vi "Create_Element_List.vi"() -> (0 "Current Element":T2, 1 "Element List":T1(array[cluster]))   [LabVIEW 2009]
panel:
  in  "String":string
  in  "Charakters_Cluster":T3={"Initial position"=[24.39, -7.31], "interval of charactors (Y)\n\"-\"down; \"+\" up"=0.0, "interval of charactors (X)\n\"-\" right; \"+\" left"=-0.7, "change size factor\nheight=1mm*factor\nwidth=0.5mm*factor"=1.0, "String of machining charactors"="", "XY Line Arc trj"={"Velocity (units/s)"=3.0, "Acceleration (unts/s2)"=50.0, "Number of times of execution"=1}} {"XY Line Arc trj"."Acceleration (unts/s2)" format="%.6f"; "XY Line Arc trj"."Velocity (units/s)" format="%.6f"; "XY Line Arc trj"."Number of times of execution" format="%.6f"; "Initial position" format="%.6f"}
  in  "Elektrode_Hole_Cluster":T4={"IR"=0.0, "Center of the hole  from left edge"=9.9, "Center of the hole from bottom edge"=2.35, "OR"=0.4, "ablation rate"=0.01, "change of radus"=0.01, "Depth of the hole"=4.0, "XY Line Arc Trajectory"={"Velocity (units/s)"=0.5, "Acceleration (unts/s2)"=20.0, "Number of times of execution"=1}} {"XY Line Arc Trajectory"."Acceleration (unts/s2)" format="%.6f"; "XY Line Arc Trajectory"."Velocity (units/s)" format="%.6f"; "XY Line Arc Trajectory"."Number of times of execution" format="%.6f"}
  in  "Gas_Jet_Cluster":T5={"Hight to groove(tube center)"=3.0, "Origin to jet outlet (Jet toal)"=10.0, "Laser interval tube"=0.01, "Ab rate tube"=0.016, "Machining geometry (mm)"={"a0 radius"=0.35, "a0 depth"=0.5, "b0 radius"=0.1, "b0(depth)"=0.15, "a1 radius"=0.2, "a1 depth"=0.3}, "Gap between  \nl1 and l2 "=0.003, "Length"={" l0"=0.5, "l1"=0.35, "l 2"=0.5, "l 3"=0.5}, "Laser interval jet"=0.008, "Ab rate jet"=0.01, "XY Line Arc Trajectory jet"={"Velocity (units/s)"=3.0, "Acceleration (unts/s2)"=20.0, "Number of times of execution"=1}, "XY Line Arc Trajectory tube"={"Velocity (units/s)"=3.0, "Acceleration (unts/s2)"=20.0, "Number of times of execution"=1}} {"XY Line Arc Trajectory tube"."Acceleration (unts/s2)" format="%.6f"; "XY Line Arc Trajectory tube"."Velocity (units/s)" format="%.6f"; "XY Line Arc Trajectory tube"."Number of times of execution" format="%.6f"; "XY Line Arc Trajectory jet"."Acceleration (unts/s2)" format="%.6f"; "XY Line Arc Trajectory jet"."Velocity (units/s)" format="%.6f"; "XY Line Arc Trajectory jet"."Number of times of execution" format="%.6f"}
  in  "Curved_Slot_Cluster":T6={"X distance from left edge"=10.5, "Height to groove"=2.5, "Remove distance"=3.5, "a0 radius"=0.9, "ablation rate"=0.01, "interval between laser path"=0.01, "Length "=11.0, "XY Line Arc Trajectory part 1"={"Velocity (units/s)"=3.0, "Acceleration (unts/s2)"=20.0, "Number of times of execution"=1}, "Slot geometry"={FALSE, FALSE}} {"XY Line Arc Trajectory part 1"."Acceleration (unts/s2)" format="%.6f"; "XY Line Arc Trajectory part 1"."Velocity (units/s)" format="%.6f"; "XY Line Arc Trajectory part 1"."Number of times of execution" format="%.6f"}
  in  "Cap_cluster":T7={"Height to cap"=3.0, "Interval of  laser path"=0.008, "Ab rate"=0.005, "Radus of Cap "=0.1, "Length of Cap"=3.0, "XY Line Arc Trajectory part 1"={"Velocity (units/s)"=3.0, "Acceleration (unts/s2)"=20.0, "Number of times of execution"=1}} {"XY Line Arc Trajectory part 1"."Acceleration (unts/s2)" format="%.6f"; "XY Line Arc Trajectory part 1"."Velocity (units/s)" format="%.6f"; "XY Line Arc Trajectory part 1"."Number of times of execution" format="%.6f"}
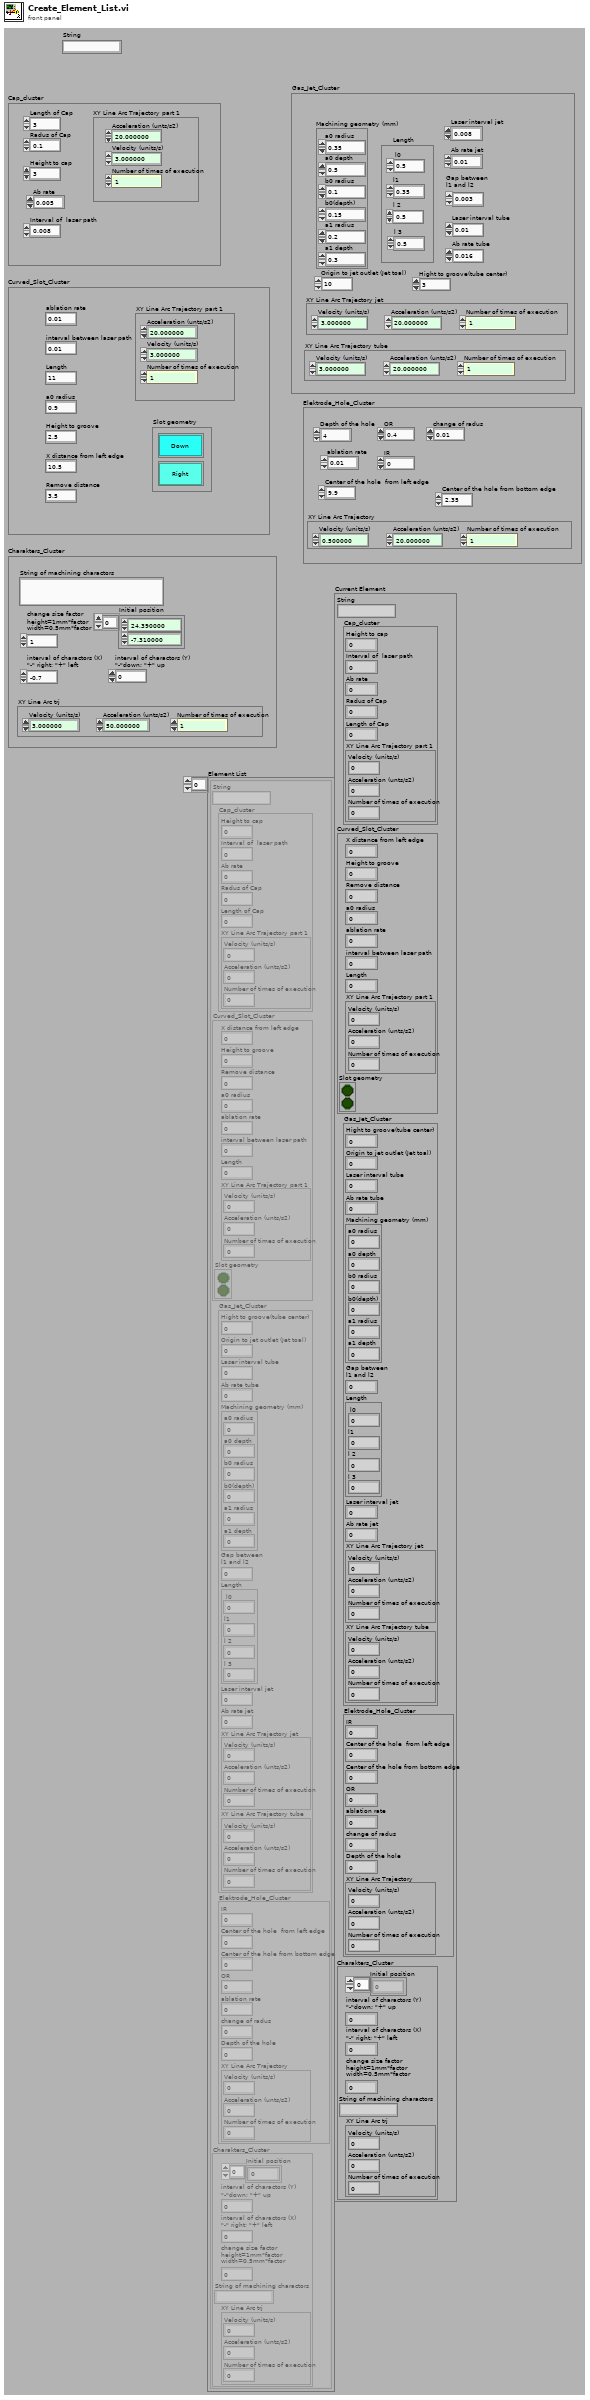
[diagram p1: front panel]
types:
  T1 = cluster{"String":string, "Cap_cluster":cluster{"Height to cap":dbl, "Interval of  laser path":dbl, "Ab rate":dbl, "Radus of Cap ":dbl, "Length of Cap":dbl, "XY Line Arc Trajectory part 1":cluster{"Velocity (units/s)":dbl, "Acceleration (unts/s2)":dbl, "Number of times of execution":i32}}, "Curved_Slot_Cluster":cluster{"X distance from left edge":dbl, "Height to groove":dbl, "Remove distance":dbl, "a0 radius":dbl, "ablation rate":dbl, "interval between laser path":dbl, "Length ":dbl, "XY Line Arc Trajectory part 1":cluster{"Velocity (units/s)":dbl, "Acceleration (unts/s2)":dbl, "Number of times of execution":i32}, "Slot geometry":cluster{bool, bool}}, "Gas_Jet_Cluster":cluster{"Hight to groove(tube center)":dbl, "Origin to jet outlet (Jet toal)":dbl, "Laser interval tube":dbl, "Ab rate tube":dbl, "Machining geometry (mm)":cluster{"a0 radius":dbl, "a0 depth":dbl, "b0 radius":dbl, "b0(depth)":dbl, "a1 radius":dbl, "a1 depth":dbl}, "Gap between  \nl1 and l2 ":dbl, "Length":cluster{" l0":dbl, "l1":dbl, "l 2":dbl, "l 3":dbl}, "Laser interval jet":dbl, "Ab rate jet":dbl, "XY Line Arc Trajectory jet":cluster{"Velocity (units/s)":dbl, "Acceleration (unts/s2)":dbl, "Number of times of execution":i32}, "XY Line Arc Trajectory tube":cluster{"Velocity (units/s)":dbl, "Acceleration (unts/s2)":dbl, "Number of times of execution":i32}}, "Elektrode_Hole_Cluster":cluster{"IR":dbl, "Center of the hole  from left edge":dbl, "Center of the hole from bottom edge":dbl, "OR":dbl, "ablation rate":dbl, "change of radus":dbl, "Depth of the hole":dbl, "XY Line Arc Trajectory":cluster{"Velocity (units/s)":dbl, "Acceleration (unts/s2)":dbl, "Number of times of execution":i32}}, "Charakters_Cluster":cluster{"Initial position":dbl[], "interval of charactors (Y)\n\"-\"down; \"+\" up":dbl, "interval of charactors (X)\n\"-\" right; \"+\" left":dbl, "change size factor\nheight=1mm*factor\nwidth=0.5mm*factor":dbl, "String of machining charactors":string, "XY Line Arc trj":cluster{"Velocity (units/s)":dbl, "Acceleration (unts/s2)":dbl, "Number of times of execution":i32}}}[]
  T2 = cluster{"String":string, "Cap_cluster":cluster{"Height to cap":dbl, "Interval of  laser path":dbl, "Ab rate":dbl, "Radus of Cap ":dbl, "Length of Cap":dbl, "XY Line Arc Trajectory part 1":cluster{"Velocity (units/s)":dbl, "Acceleration (unts/s2)":dbl, "Number of times of execution":i32}}, "Curved_Slot_Cluster":cluster{"X distance from left edge":dbl, "Height to groove":dbl, "Remove distance":dbl, "a0 radius":dbl, "ablation rate":dbl, "interval between laser path":dbl, "Length ":dbl, "XY Line Arc Trajectory part 1":cluster{"Velocity (units/s)":dbl, "Acceleration (unts/s2)":dbl, "Number of times of execution":i32}, "Slot geometry":cluster{bool, bool}}, "Gas_Jet_Cluster":cluster{"Hight to groove(tube center)":dbl, "Origin to jet outlet (Jet toal)":dbl, "Laser interval tube":dbl, "Ab rate tube":dbl, "Machining geometry (mm)":cluster{"a0 radius":dbl, "a0 depth":dbl, "b0 radius":dbl, "b0(depth)":dbl, "a1 radius":dbl, "a1 depth":dbl}, "Gap between  \nl1 and l2 ":dbl, "Length":cluster{" l0":dbl, "l1":dbl, "l 2":dbl, "l 3":dbl}, "Laser interval jet":dbl, "Ab rate jet":dbl, "XY Line Arc Trajectory jet":cluster{"Velocity (units/s)":dbl, "Acceleration (unts/s2)":dbl, "Number of times of execution":i32}, "XY Line Arc Trajectory tube":cluster{"Velocity (units/s)":dbl, "Acceleration (unts/s2)":dbl, "Number of times of execution":i32}}, "Elektrode_Hole_Cluster":cluster{"IR":dbl, "Center of the hole  from left edge":dbl, "Center of the hole from bottom edge":dbl, "OR":dbl, "ablation rate":dbl, "change of radus":dbl, "Depth of the hole":dbl, "XY Line Arc Trajectory":cluster{"Velocity (units/s)":dbl, "Acceleration (unts/s2)":dbl, "Number of times of execution":i32}}, "Charakters_Cluster":cluster{"Initial position":dbl[], "interval of charactors (Y)\n\"-\"down; \"+\" up":dbl, "interval of charactors (X)\n\"-\" right; \"+\" left":dbl, "change size factor\nheight=1mm*factor\nwidth=0.5mm*factor":dbl, "String of machining charactors":string, "XY Line Arc trj":cluster{"Velocity (units/s)":dbl, "Acceleration (unts/s2)":dbl, "Number of times of execution":i32}}}
  T3 = cluster{"Initial position":dbl[], "interval of charactors (Y)\n\"-\"down; \"+\" up":dbl, "interval of charactors (X)\n\"-\" right; \"+\" left":dbl, "change size factor\nheight=1mm*factor\nwidth=0.5mm*factor":dbl, "String of machining charactors":string, "XY Line Arc trj":cluster{"Velocity (units/s)":dbl, "Acceleration (unts/s2)":dbl, "Number of times of execution":i32}}
  T4 = cluster{"IR":dbl, "Center of the hole  from left edge":dbl, "Center of the hole from bottom edge":dbl, "OR":dbl, "ablation rate":dbl, "change of radus":dbl, "Depth of the hole":dbl, "XY Line Arc Trajectory":cluster{"Velocity (units/s)":dbl, "Acceleration (unts/s2)":dbl, "Number of times of execution":i32}}
  T5 = cluster{"Hight to groove(tube center)":dbl, "Origin to jet outlet (Jet toal)":dbl, "Laser interval tube":dbl, "Ab rate tube":dbl, "Machining geometry (mm)":cluster{"a0 radius":dbl, "a0 depth":dbl, "b0 radius":dbl, "b0(depth)":dbl, "a1 radius":dbl, "a1 depth":dbl}, "Gap between  \nl1 and l2 ":dbl, "Length":cluster{" l0":dbl, "l1":dbl, "l 2":dbl, "l 3":dbl}, "Laser interval jet":dbl, "Ab rate jet":dbl, "XY Line Arc Trajectory jet":cluster{"Velocity (units/s)":dbl, "Acceleration (unts/s2)":dbl, "Number of times of execution":i32}, "XY Line Arc Trajectory tube":cluster{"Velocity (units/s)":dbl, "Acceleration (unts/s2)":dbl, "Number of times of execution":i32}}
  T6 = cluster{"X distance from left edge":dbl, "Height to groove":dbl, "Remove distance":dbl, "a0 radius":dbl, "ablation rate":dbl, "interval between laser path":dbl, "Length ":dbl, "XY Line Arc Trajectory part 1":cluster{"Velocity (units/s)":dbl, "Acceleration (unts/s2)":dbl, "Number of times of execution":i32}, "Slot geometry":cluster{bool, bool}}
  T7 = cluster{"Height to cap":dbl, "Interval of  laser path":dbl, "Ab rate":dbl, "Radus of Cap ":dbl, "Length of Cap":dbl, "XY Line Arc Trajectory part 1":cluster{"Velocity (units/s)":dbl, "Acceleration (unts/s2)":dbl, "Number of times of execution":i32}}
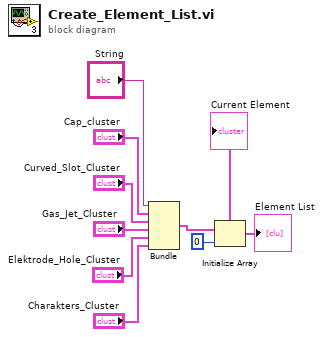
[diagram p0: block diagram]
diagram:
  n1 = Bundle("String"="String", "Cap_cluster"="Cap_cluster", "Curved_Slot_Cluster"="Curved_Slot_Cluster", "Gas_Jet_Cluster"="Gas_Jet_Cluster", "Elektrode_Hole_Cluster"="Elektrode_Hole_Cluster", "Charakters_Cluster"="Charakters_Cluster") -> (w2:T2)  [unwired: 1 in]
  "Current Element" <- w2
  n2 = Initialize Array(w2, 0 ("dimension size")) -> (→"Element List":T1)
